vi "mlink_ao_scan_data.vi"(6 "channels":u8[](array[numeric]), 7 "opt":T1(ring), 8 "error in (no error)":errorcluster, 10 "data":sgl[](array[numeric]), 11 "connection ID":i32=-1) -> (0 "error out":errorcluster, 3 "connection ID out":i32)   [LabVIEW 2009, in "MicroDAQ.lvlib" / "mlink.lvlib"]
doc: "This function queues data to be output. A function call has to be preceded with\nmlink_ao_scan_init() . Function queues data in the stream and periodic mode and its behavior\ndepends on selected scan mode. In periodic mode, the function can queue data for every\nchannel combination from used channels (defined in mlink_ao_scan_init() ). If e.g. in\nscanning session four channels are used: 1, 2, 3, 4 mlink_ao_scan_data() can be called to\nqueue data for 1 or 4 or 1,2 or 1,4, or 3,4 etc. channel or queue data for all selected channels.\nIn periodic mode channels argument can contain every combination of used channels, while in\nstream mode channel argument must be the same as used in mlink_ao_scan_init() . The data\nargument in stream mode must have the same size as the data argument in function\nmlink_ao_scan_init() . The mlink_ao_scan_init() perform initial data queue operation. The\nperiodic mode uses a single buffer which data is output from. When the end of the buffer is\nreached, data index is switched to the beginning of the buffer. The mlink_ao_scan_data()\nfunction overwrites the whole buffer with new data. Depending on the scanning mode opt\nargument has a different meaning. When the periodic mode is used opt argument allows\ncontrolling data index after queuing data. When opt=1 data index will be set to the beginning\nof the buffer. If opt=0 queue operation doesn't affect data index."
uses:
  <instrlib>/MicroDAQ/Mlink library wraper/mlink.lvlib
  <instrlib>/MicroDAQ/MLink32.dll
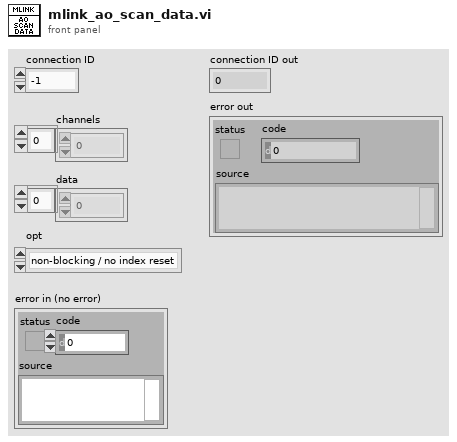
[diagram p1: front panel]
types:
  T1 = enum8{"non-blocking / no index reset", "blocking / index reset"}
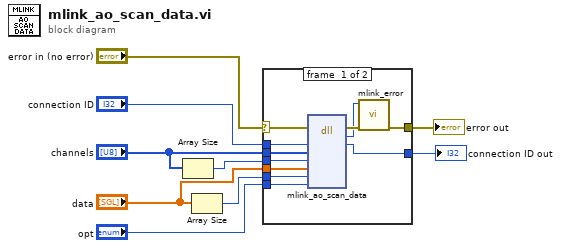
[diagram p0: block diagram]
diagram:
  n1 = Array Size(array="channels") -> (size(s)=w6:i32)
  n2 = Array Size(array="data") -> (size(s)=w2:i32)
  n3 = case shown="No Error" "error in (no error)" {
    selector: "error in (no error)" -> [w18 w22]
    tunnel: "connection ID" -> [w20 w21]
    tunnel: [w19 w21] -> w8
    tunnel: w6 -> [w17 _]
    tunnel: "opt" -> [w16 _]
    tunnel: "channels" -> [w15 _]
    tunnel: "data" -> [w14 _]
    tunnel: w2 -> [w13 _]
    tunnel: [w10 w22] -> w1
    frame #0 {
      n4 = dll-call lib="C:/Program Files (x86)/National Instruments/LabVIEW 2009/instr.lib/MicroDAQ/MLink32.dll" fn="mlink_ao_scan_data"(error in=w18, "connection ID"=w20, "channels"=w15, "count"=w17, "data"=w14, "data_size"=w13, "opt"=w16) -> (error out=w12:errorcluster, "return type"=w11:i32, "connection ID"=w19:i32)  [unwired: 7 in, 1 out]
      n5 = call <instrlib>:"mlink_error.vi"("error in (no error)"=w12, "error code"=w11) -> ("error out"=w10:errorcluster)  [unwired: 9 in]
    }
    frame #1 {
    }
  }
  "connection ID out" <- w8
  "error out" <- w1
